vi "Check_Http.vi"(3 "error in (no error)":errorcluster, 4 "StartLotTraveler In":T1, 5 "LotData in":refnum<class "LotData.lvclass">) -> (0 "error out":errorcluster, 1 "StartLotTraveler Out":T1, 2 "LotData out":refnum<class "LotData.lvclass">)   [LabVIEW 2012, in "LotData.lvclass"]
uses:
  Classes/LotData.lvclass
  Controls/StartLotTraveler.ctl
  Controls/MeasurementType.ctl
  Controls/ProbeStationId.vi
  <vilib>/LVH/i3 JSON/JSON Parsing/Get Object Parameter Files/Get Object Parameter - Boolean.vi
  <vilib>/LVH/i3 JSON/JSON Parsing/Get Object Parameter Files/Get Object Parameter - Numeric.vi
  <vilib>/httpClient/LabVIEWHTTPClient.lvlib
  <vilib>/LVH/i3 JSON/i3-json.lvlib
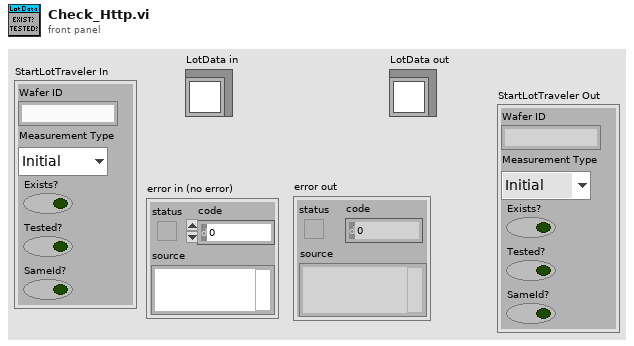
[diagram p1: front panel]
types:
  T1 = typedef "StartLotTraveler.ctl" = cluster{"Wafer ID":string, "Measurement Type":T2, "Exists?":bool, "Tested?":bool, "SameId?":bool}
  T2 = typedef "MeasurementType.ctl" = enum16{"Initial", "Final"}
  T3 = typedef "LabVIEWHTTPClient.lvlib/ClientHandle.ctl" = refnum<k1>
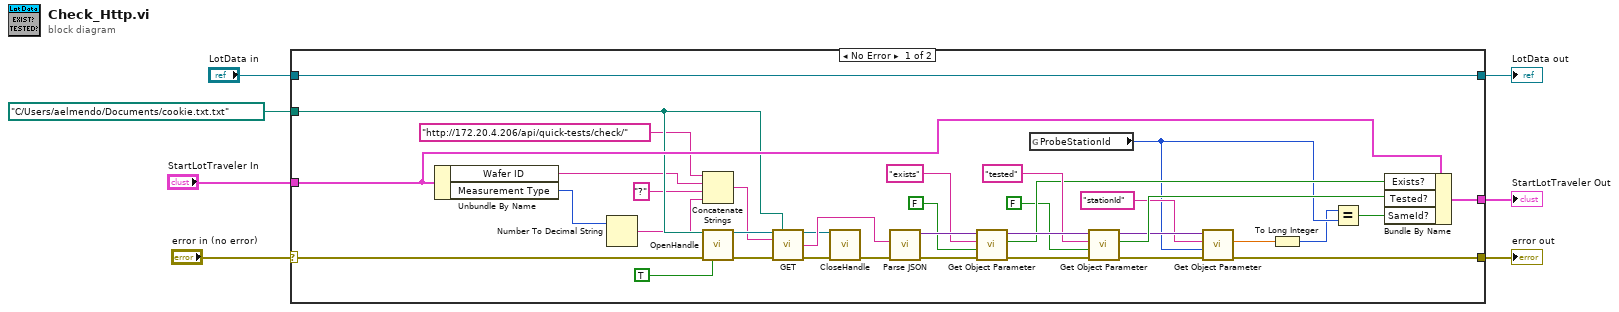
[diagram p0: block diagram]
diagram:
  n1 = case shown="No Error" "error in (no error)" {
    selector: "error in (no error)" -> [w8 w46]
    tunnel: [w9 w46] -> w7
    tunnel: [w43 w45] -> w6
    tunnel: "LotData in" -> [w43 w45]
    tunnel: "StartLotTraveler In" -> [w42 w44]
    tunnel: [w40 w44] -> w2
    tunnel: path "C:/Users/aelmendo/Documents/cookie.txt.txt" ("output file") -> [w36 _]
    frame No Error {
      n2 = Unbundle By Name(w42) -> ("Wafer ID"=w14:string, "Measurement Type"=w12:T2)
      n3 = Number To Decimal String(number=w12) -> (decimal integer string=w11:string)  [unwired: 1 in]
      n4 = Concatenate Strings("http://172.20.4.206/api/quick-tests/check/" ("url"), w14, "?" ("string"), w11) -> (w10:string)
      n5 = call <vilib>:"OpenHandle.vi"("cookie file"=w36, "error in (no error)"=w8, "verify server(true)"=TRUE) -> ("client handle out"=w39:T3, "error out"=w38:errorcluster)  [unwired: 11 in]
      n6 = call <vilib>:"GET.vi"("client handle"=w39, "output file"=w36, "url"=w10, "error in (no error)"=w38) -> ("client handle out"=w34:T3, "body"=w35:string, "error out"=w33:errorcluster)  [unwired: 8 in, 1 out]
      n7 = call <vilib>:"CloseHandle.vi"("client handle"=w34, "error in (no error)"=w33) -> ("error out"=w32:errorcluster)  [unwired: 13 in]
      n8 = call <vilib>:"Parse JSON.vi"("error in (no error)"=w32, "JSON String"=w35) -> ("error out"=w27:errorcluster, "JSON Tree"=w31:variant)  [unwired: 6 in, 2 out]
      n9 = call-poly <vilib>:"Get Object Parameter.vi"("error in (no error)"=w27, "Default Value if JSON Null"=FALSE, "Parameter Name"="exists", "JSON Tree In (JSON Object)"=w31) -> ("error out"=w28:errorcluster, "Boolean Value"=w23:bool, "JSON Tree Out Passthrough"=w29:variant)  [unwired: 4 in, 1 out]
      n10 = global read "ProbeStationId.vi" "ProbeStationId"() -> (w18:i32)
      n11 = call-poly <vilib>:"Get Object Parameter.vi"("error in (no error)"=w28, "Default Value if JSON Null"=FALSE, "Parameter Name"="tested", "JSON Tree In (JSON Object)"=w29) -> ("error out"=w20:errorcluster, "Boolean Value"=w24:bool, "JSON Tree Out Passthrough"=w22:variant)  [unwired: 4 in, 1 out]
      n12 = call-poly <vilib>:"Get Object Parameter.vi"("error in (no error)"=w20, "Default Value if JSON Null"=w18, "Parameter Name"="stationId", "JSON Tree In (JSON Object)"=w22) -> ("error out"=w9:errorcluster, "Double Value"=w17:dbl)  [unwired: 4 in, 2 out]
      n13 = To Long Integer(number=w17) -> (32bit integer=w16:i32)
      n14 = Equal?(x=w16, y=w18) -> (x = y?=w41:bool)
      n15 = Bundle By Name(cluster=w42, "Exists?"=w23, "Tested?"=w24, "SameId?"=w41) -> (w40:T1)
    }
    frame Error {
    }
  }
  "error out" <- w7
  "LotData out" <- w6
  "StartLotTraveler Out" <- w2
